vi "Gyro Before Enable Calibrator.vi"(8 "error in":errorcluster, 11 "Sensors":T1={"Gyro"={"DevStatus"={"status"=FALSE, "code"=0, "source"=""}, "Analog Module"=enum."Controller 1", "Analog Channel"=enum."AI 0", "Offset"=0.0, "Gain (VoltsPerDegree/Second)"=0.0}, "Encoders"={"Left Drive CAN"={"DeviceStatus"={"status"=FALSE, "code"=0, "source"=""}, "Type"=enum."PWM", "PWM"={"Controller"=enum."Controller 1", "PWM Channel"=enum."PWM 0", "DeadBand"={"Name"="", "maxPositivePwm"=0, "minPositivePwm"=0, "centerPwm"=0, "maxNegativePwm"=0, "minNegativePwm"=0, "angularRange"=0}}, "CAN"={"Device Number"=0, "Control Mode"=enum."Percent VBus", "Semaphore"=refnum, "Max Vout"=0.0, "TalonSRX Control Mode"=enum."Percent VBus"}, "Invert"=FALSE, "TransformRef"=refnum, "InvTransformRef"=refnum}, "Right Drive CAN"={"DeviceStatus"={"status"=FALSE, "code"=0, "source"=""}, "Type"=enum."PWM", "PWM"={"Controller"=enum."Controller 1", "PWM Channel"=enum."PWM 0", "DeadBand"={"Name"="", "maxPositivePwm"=0, "minPositivePwm"=0, "centerPwm"=0, "maxNegativePwm"=0, "minNegativePwm"=0, "angularRange"=0}}, "CAN"={"Device Number"=0, "Control Mode"=enum."Percent VBus", "Semaphore"=refnum, "Max Vout"=0.0, "TalonSRX Control Mode"=enum."Percent VBus"}, "Invert"=FALSE, "TransformRef"=refnum, "InvTransformRef"=refnum}, "Strafe CAN"={"DeviceStatus"={"status"=FALSE, "code"=0, "source"=""}, "Type"=enum."PWM", "PWM"={"Controller"=enum."Controller 1", "PWM Channel"=enum."PWM 0", "DeadBand"={"Name"="", "maxPositivePwm"=0, "minPositivePwm"=0, "centerPwm"=0, "maxNegativePwm"=0, "minNegativePwm"=0, "angularRange"=0}}, "CAN"={"Device Number"=0, "Control Mode"=enum."Percent VBus", "Semaphore"=refnum, "Max Vout"=0.0, "TalonSRX Control Mode"=enum."Percent VBus"}, "Invert"=FALSE, "TransformRef"=refnum, "InvTransformRef"=refnum}, "Elevator CAN"={"DeviceStatus"={"status"=FALSE, "code"=0, "source"=""}, "Type"=enum."PWM", "PWM"={"Controller"=enum."Controller 1", "PWM Channel"=enum."PWM 0", "DeadBand"={"Name"="", "maxPositivePwm"=0, "minPositivePwm"=0, "centerPwm"=0, "maxNegativePwm"=0, "minNegativePwm"=0, "angularRange"=0}}, "CAN"={"Device Number"=0, "Control Mode"=enum."Percent VBus", "Semaphore"=refnum, "Max Vout"=0.0, "TalonSRX Control Mode"=enum."Percent VBus"}, "Invert"=FALSE, "TransformRef"=refnum, "InvTransformRef"=refnum}}, "Switches"={"Elevator Top"={"DevStatus"={"status"=FALSE, "code"=0, "source"=""}, "DIO Channel"=enum."DIO 0", "Controller"=enum."Controller 1", "CntIndex"=enum."Ctr 0", "Normally Closed"=FALSE}, "Elevator Bottom"={"DevStatus"={"status"=FALSE, "code"=0, "source"=""}, "DIO Channel"=enum."DIO 0", "Controller"=enum."Controller 1", "CntIndex"=enum."Ctr 0", "Normally Closed"=FALSE}, "Claw Outside"={"DevStatus"={"status"=FALSE, "code"=0, "source"=""}, "DIO Channel"=enum."DIO 0", "Controller"=enum."Controller 1", "CntIndex"=enum."Ctr 0", "Normally Closed"=FALSE}, "Tote Touch"={"DevStatus"={"status"=FALSE, "code"=0, "source"=""}, "DIO Channel"=enum."DIO 1", "Controller"=enum."Controller 1", "CntIndex"=enum."Invalid", "Normally Closed"=FALSE}}, "Arm Capper Pot"={"DevStatus"={"status"=FALSE, "code"=0, "source"=""}, "Controller"=enum."Controller 1", "Analog Channel"=enum."AI 0", "Invert Output"=FALSE}, "Arm Angle Pot"={"DevStatus"={"status"=FALSE, "code"=0, "source"=""}, "Controller"=enum."Controller 1", "Analog Channel"=enum."AI 0", "Invert Output"=FALSE}, "Sonar"={"Front"={"AIDeviceRef"={"DevStatus"={"status"=FALSE, "code"=0, "source"=""}, "Controller"=enum."Controller 1", "Analog Channel"=enum."Invalid"}, "Scaling factor (V/in)"=0.0098, "Average Bits"=3}, "Back"={"AIDeviceRef"={"DevStatus"={"status"=FALSE, "code"=0, "source"=""}, "Controller"=enum."Controller 1", "Analog Channel"=enum."Invalid"}, "Scaling factor (V/in)"=0.0098, "Average Bits"=3}}} {"Sonar"."Back"."Average Bits" max=15; "Sonar"."Front"."Average Bits" max=15}) -> ()   [LabVIEW 2014]
uses:
  Utilities/Sensors.ctl
  <vilib>/Rock Robotics/WPI/Gyro/WPI_GyroDevRef.ctl
  <vilib>/Rock Robotics/SystemInterfaces/Typedef/FPGA_TypedefAnalogModule.ctl
  <vilib>/Rock Robotics/SystemInterfaces/AI/FPGA_AIChannel.ctl
  <vilib>/Rock Robotics/WPI/MotorControl/WPI_MotorControlDeviceRef.ctl
  <vilib>/Rock Robotics/WPI/MotorControl/WPI_MotorControlType.ctl
  <vilib>/Rock Robotics/SystemInterfaces/Typedef/FPGA_TypedefDigitalModule.ctl
  <vilib>/Rock Robotics/SystemInterfaces/DIO/FPGA_DIOPWMChannel.ctl
  <vilib>/Rock Robotics/WPI/PWM/WPI_PWMDeadband.ctl
  <vilib>/Rock Robotics/WPI/CAN/Jaguar/SubVIs/WPI_CANJaguar_ControlMode.ctl
  <vilib>/Rock Robotics/WPI/CAN/TalonSRX/WPI_CANTalonSRX_APIControlMode.ctl
  <vilib>/Rock Robotics/WPI/PWM/WPI_PWMTransform_ConPane.ctl
  <vilib>/Rock Robotics/WPI/Switch/WPI_SwitchDevRef.ctl
  <vilib>/Rock Robotics/SystemInterfaces/DIO/FPGA_DIOChannel.ctl
  <vilib>/Rock Robotics/SystemInterfaces/Counter/FPGA_CounterCtrSystemIndex.ctl
  <vilib>/Rock Robotics/WPI/Potentiometer/WPI_PotentiometerDevRef.ctl
  <vilib>/Rock Robotics/WPI/Ultrasonic/WPI_SonarMB1010AnalogDeviceRef.ctl
  <vilib>/Rock Robotics/WPI/AnalogChannel/WPI_AnalogChannelDevRef.ctl
  <vilib>/Rock Robotics/WPI/DriverStation/WPI_DriverStationRobotMode2.ctl
  <vilib>/Rock Robotics/SystemInterfaces/AI/FPGA_AIDevRef.ctl
  Main/Robot Global Data.vi
panel:
  in  "Calibration Time (s)":dbl=1.0
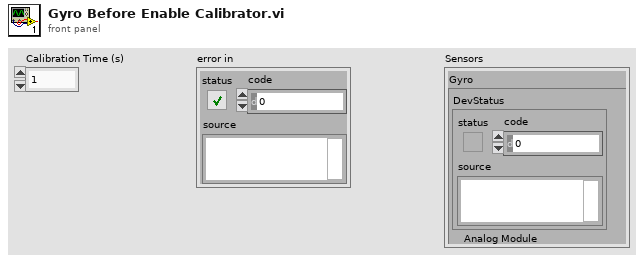
[diagram p1: front panel]
types:
  T1 = typedef "Sensors.ctl" = cluster{"Gyro":T2, "Encoders":cluster{"Left Drive CAN":T5, "Right Drive CAN":T5, "Strafe CAN":T5, "Elevator CAN":T5}, "Switches":cluster{"Elevator Top":T14, "Elevator Bottom":T14, "Claw Outside":T14, "Tote Touch":T14}, "Arm Capper Pot":T17, "Arm Angle Pot":T17, "Sonar":cluster{"Front":T18, "Back":T18}}
  T2 = typedef "WPI_GyroDevRef.ctl" = cluster{"DevStatus":errorcluster, "Analog Module":T3, "Analog Channel":T4, "Offset":dbl, "Gain (VoltsPerDegree/Second)":dbl}
  T3 = typedef "FPGA_TypedefAnalogModule.ctl" = enum16{"Controller 1"}
  T4 = typedef "FPGA_AIChannel.ctl" = enum8{"AI 0", "AI 1", "AI 2", "AI 3", "AI MXP 0", "AI MXP 1", "AI MXP 2", "AI MXP 3", "Invalid"}
  T5 = typedef "WPI_MotorControlDeviceRef.ctl" = cluster{"DeviceStatus":errorcluster, "Type":T6, "PWM":cluster{"Controller":T7, "PWM Channel":T8, "DeadBand":T9}, "CAN":cluster{"Device Number":u8, "Control Mode":T10, "Semaphore":T11, "Max Vout":dbl, "TalonSRX Control Mode":T12}, "Invert":bool, "TransformRef":T13, "InvTransformRef":T13}
  T6 = typedef "WPI_MotorControlType.ctl" = enum16{"PWM", "CAN", "CANTalonSRX"}
  T7 = typedef "FPGA_TypedefDigitalModule.ctl" = enum16{"Controller 1"}
  T8 = typedef "FPGA_DIOPWMChannel.ctl" = enum8{"PWM 0", "PWM 1", "PWM 2", "PWM 3", "PWM 4", "PWM 5", "PWM 6", "PWM 7", "PWM 8", "PWM 9", "PWM MXP 0", "PWM MXP 1", "PWM MXP 2", "PWM MXP 3", "PWM MXP 4", "PWM MXP 5", "PWM MXP 6", "PWM MXP 7", "PWM MXP 8", "PWM MXP 9", "Invalid"}
  T9 = typedef "WPI_PWMDeadband.ctl" = cluster{"Name":string, "maxPositivePwm":i32, "minPositivePwm":i32, "centerPwm":i32, "maxNegativePwm":i32, "minNegativePwm":i32, "angularRange":u16}
  T10 = typedef "WPI_CANJaguar_ControlMode.ctl" = enum8{"Percent VBus", "Current", "Speed", "Position", "Voltage"}
  T11 = typedef "Semaphore RefNum" = refnum<k1>
  T12 = typedef "WPI_CANTalonSRX_APIControlMode.ctl" = enum8{"Percent VBus", "Speed", "Position", "Slave", "Unchanged / Invalid"}
  T13 = typedef "WPI_PWMTransform_ConPane.ctl" = refnum<vi>
  T14 = typedef "WPI_SwitchDevRef.ctl" = cluster{"DevStatus":errorcluster, "DIO Channel":T15, "Controller":T7, "CntIndex":T16, "Normally Closed":bool}
  T15 = typedef "FPGA_DIOChannel.ctl" = enum8{"DIO 0", "DIO 1", "DIO 2", "DIO 3", "DIO 4", "DIO 5", "DIO 6", "DIO 7", "DIO 8", "DIO 9", "DIO MXP 0", "DIO MXP 1", "DIO MXP 2", "DIO MXP 3", "DIO MXP 4", "DIO MXP 5", "DIO MXP 6", "DIO MXP 7", "DIO MXP 8", "DIO MXP 9", "DIO MXP 10", "DIO MXP 11", "DIO MXP 12", "DIO MXP 13", "DIO MXP 14", "DIO MXP 15", "Invalid"}
  T16 = typedef "FPGA_CounterCtrSystemIndex.ctl" = enum8{"Ctr 0", "Ctr 1", "Ctr 2", "Ctr 3", "Ctr 4", "Ctr 5", "Ctr 6", "Ctr 7", "Invalid"}
  T17 = typedef "WPI_PotentiometerDevRef.ctl" = cluster{"DevStatus":errorcluster, "Controller":T3, "Analog Channel":T4, "Invert Output":bool}
  T18 = typedef "WPI_SonarMB1010AnalogDeviceRef.ctl" = cluster{"AIDeviceRef":T19, "Scaling factor (V/in)":dbl, "Average Bits":u8}
  T19 = typedef "WPI_AnalogChannelDevRef.ctl" = cluster{"DevStatus":errorcluster, "Controller":T3, "Analog Channel":T4}
  T20 = typedef "WPI_DriverStationRobotMode2.ctl" = enum16{"Autonomous Disabled", "Autonomous Enabled", "Teleop Disabled", "Teleop Enabled", "Disconnected", "Finish", "Test Disabled", "Test Enabled", "Emergency Stopped"}
  T21 = typedef "FPGA_AIDevRef.ctl" = cluster{"DevStatus":errorcluster, "Controller":T3}
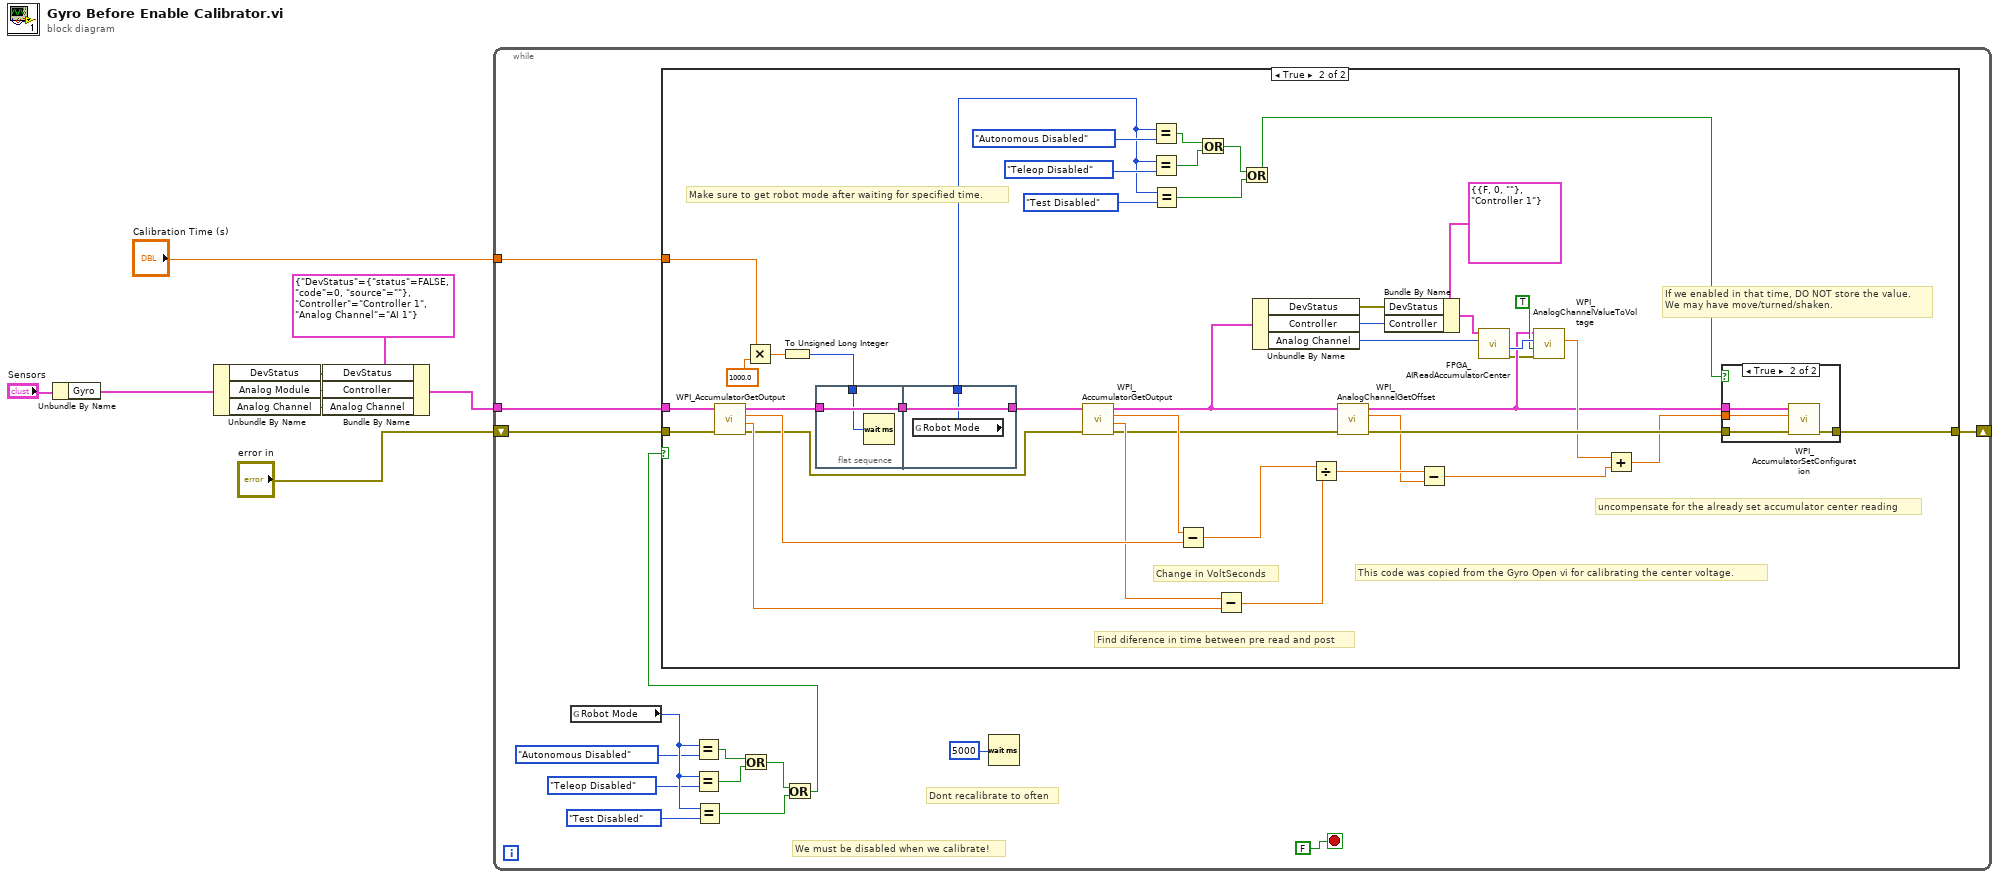
[diagram p0: block diagram]
diagram:
  n1 = Unbundle By Name("Sensors") -> ("Gyro"=w1:T2)
  n2 = Unbundle By Name(w1) -> ("DevStatus"=w8:errorcluster, "Analog Module"=w7:T3, "Analog Channel"=w6:T4)
  n3 = Bundle By Name(cluster=T19 {"DevStatus"={"status"=FALSE, "code"=0, "source"=""}, "Controller"=enum."Controller 1", "Analog Channel"=enum."AI 1"} ("AIDeviceRef"), "DevStatus"=w8, "Controller"=w7, "Analog Channel"=w6) -> (w4:T19)
  n4 = while {
    tunnel: "Calibration Time (s)" -> [w23]
    tunnel: w4 -> [w24]
    shift-right: [w22] -> _
    shift-left: "error in" -> [w21]
    stop <- FALSE stop-if-true
    # "We must be disabled when we calibrate!"
    # "Dont recalibrate to often"
    n5 = global read "Robot Global Data.vi" "Robot Mode"() -> (w19:T20)
    n6 = Equal?(x=w19, y=WPI_DriverStationRobotMode2."Autonomous Disabled" ("Robot Mode")) -> (x = y?=w15:bool)
    n7 = Equal?(x=w19, y=WPI_DriverStationRobotMode2."Teleop Disabled" ("Robot Mode")) -> (x = y?=w14:bool)
    n8 = Equal?(x=w19, y=WPI_DriverStationRobotMode2."Test Disabled" ("Robot Mode")) -> (x = y?=w13:bool)
    n9 = Or(x=w15, y=w14) -> (x .or. y?=w12:bool)
    n10 = Or(x=w12, y=w13) -> (x .or. y?=w11:bool)
    n11 = case shown="True" w11 {
      tunnel: w23 -> [_ w68]
      tunnel: w24 -> [_ w51]
      tunnel: [w25 w39] -> w22
      tunnel: w21 -> [w25 w52]
      frame False {
      }
      frame True {
        # "uncompensate for the already set accumulator center reading"
        # "Change in VoltSeconds"
        # "Find diference in time between pre read and post"
        # "Make sure to get robot mode after waiting for specified time."
        # "This code was copied from the Gyro Open vi for calibrating the center voltage."
        # "If we enabled in that time, DO NOT store the value.\nWe may have move/turned/shaken."
        n12 = call <vilib>:"WPI_AccumulatorGetOutput.vi"("error in (no error)"=w52, "AIDeviceRef"=w51) -> ("error out"=w41:errorcluster, "Duration (Seconds)"=w50:dbl, "Value (Volt Seconds)"=w49:dbl, "AIDeviceRef"=w53:T19)  [unwired: 6 out]
        n13 = Multiply(x=w68, y=1000.0) -> (x*y=w65:dbl)
        n14 = To Unsigned Long Integer(number=w65) -> (unsigned 32bit integer=w64:u32)
        n15 = flat-sequence {
          tunnel: w53 -> [w75]
          tunnel: w64 -> [w74]
          tunnel: [w75] -> w55
          tunnel: [w77] -> w40
          tunnel: w55 -> [w77]
          tunnel: [w76] -> w54
          frame #0 {
            n16 = Wait (ms)(milliseconds to wait=w74) -> ()  [unwired: 1 out]
          }
          frame #1 {
            n17 = global read "Robot Global Data.vi" "Robot Mode"() -> (w76:T20)
          }
        }
        n18 = call <vilib>:"WPI_AccumulatorGetOutput.vi"("error in (no error)"=w41, "AIDeviceRef"=w40) -> ("error out"=w42:errorcluster, "Duration (Seconds)"=w46:dbl, "Value (Volt Seconds)"=w48:dbl, "AIDeviceRef"=w34:T19)  [unwired: 6 out]
        n19 = Equal?(x=w54, y=WPI_DriverStationRobotMode2."Autonomous Disabled" ("Robot Mode")) -> (x = y?=w60:bool)
        n20 = Equal?(x=w54, y=WPI_DriverStationRobotMode2."Teleop Disabled" ("Robot Mode")) -> (x = y?=w59:bool)
        n21 = Equal?(x=w54, y=WPI_DriverStationRobotMode2."Test Disabled" ("Robot Mode")) -> (x = y?=w58:bool)
        n22 = Subtract(x=w48, y=w49) -> (x-y=w47:dbl)
        n23 = Or(x=w60, y=w59) -> (x .or. y?=w57:bool)
        n24 = Subtract(x=w46, y=w50) -> (x-y=w45:dbl)
        n25 = Or(x=w57, y=w58) -> (x .or. y?=w56:bool)
        n26 = Unbundle By Name(w34) -> ("DevStatus"=w30:errorcluster, "Controller"=w29:T3, "Analog Channel"=w33:T4)
        n27 = Divide(x=w47, y=w45) -> (x/y=w67:dbl)
        n28 = call <vilib>:"WPI_AnalogChannelGetOffset.vi"("error in (no error)"=w42, "AIDeviceRef"=w34) -> ("error out"=w44:errorcluster, "Offset"=w43:dbl, "AIDeviceRef"=w35:T19)  [unwired: 7 out]
        n29 = Bundle By Name(cluster=T21 {"DevStatus"={"status"=FALSE, "code"=0, "source"=""}, "Controller"=enum."Controller 1"} ("AI Reference in"), "DevStatus"=w30, "Controller"=w29) -> (w28:T21)
        n30 = Subtract(x=w67, y=w43) -> (x-y=w27:dbl)
        n31 = call <vilib>:"FPGA_AIReadAccumulatorCenter.vi"("Channel"=w33, "AI Reference in"=w28) -> ("error out"=w32:errorcluster, "Center"=w38:i32)  [unwired: 7 in, 1 out]
        n32 = call <vilib>:"WPI_AnalogChannelValueToVoltage.vi"("error in (no error)"=w32, "Averaged"=TRUE, "Value"=w38, "AIDeviceRef"=w35) -> ("Voltage"=w37:dbl)  [unwired: 5 in, 2 out]
        n33 = Add(x=w37, y=w27) -> (x+y=w26:dbl)
        n34 = case shown="True" w56 {
          tunnel: [w69 w73] -> w39
          tunnel: w44 -> [w69 w72]
          tunnel: w26 -> [_ w70]
          tunnel: w35 -> [_ w71]
          frame False {
          }
          frame True {
            n35 = call <vilib>:"WPI_AccumulatorSetConfiguration.vi"("error in (no error)"=w72, "Center"=w70, "AIDeviceRef"=w71) -> ("error out"=w73:errorcluster)  [unwired: 2 in, 6 out]
          }
        }
      }
    }
    n36 = Wait (ms)(milliseconds to wait=u32 5000) -> ()  [unwired: 1 out]
  }
